vi "시리얼_읽기.vi"(8 "Error In":errorcluster caption="에러 입력", 10 "Read Count":u32=1000, 11 "VISA 리소스 이름":refnum<visa-resource-name>) -> (0 "Error Out":errorcluster caption="에러 출력", 2 "Response":string, 3 "VISA 리소스 이름 출력":refnum<visa-resource-name>)   [LabVIEW 2018]
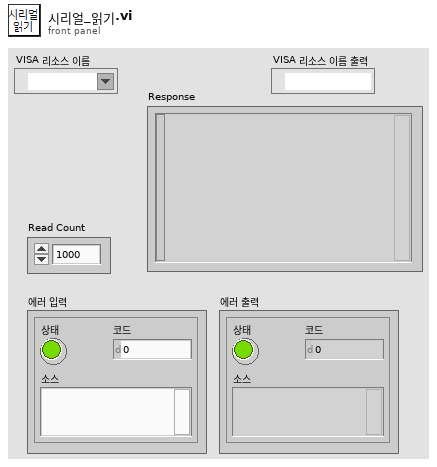
[diagram p1: front panel]
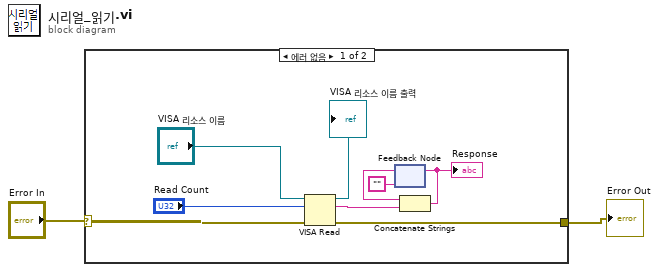
[diagram p0: block diagram]
diagram:
  n1 = case shown="에러 없음" "Error In" {
    selector: "Error In" -> [w6 _]
    tunnel: [w5 _] -> w1
    frame No Error {
      n2 = VISA Read(VISA resource name="VISA 리소스 이름", byte count="Read Count", error in (no error)=w6) -> (VISA resource name out=→"VISA 리소스 이름 출력":refnum<visa-resource-name>, read buffer=w10:string, error out=w5:errorcluster)  [unwired: 1 out]
      n3 = feedback #1("") -> (w9:string)
      n4 = Concatenate Strings(w9, w10) -> (w8:string)
      "Response" <- w8
      n5 = feedback-in #1(w8) -> ()
    }
    frame Error {
    }
  }
  "Error Out" <- w1
